vi "Remove Filename Invalid Char.vi"(2 "Input string":string, 6 "Replace Using ...":enum16{"Underscore", "Space"}(ring)) -> (16 "Output String":string)   [LabVIEW 2022 SP3, in "Generic Utilities.lvclass"]
uses:
  Generic Utilities.lvclass
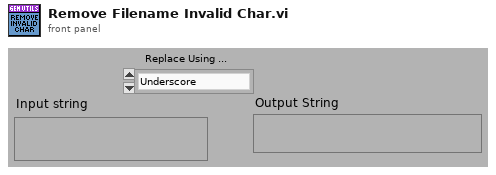
[diagram p1: front panel]
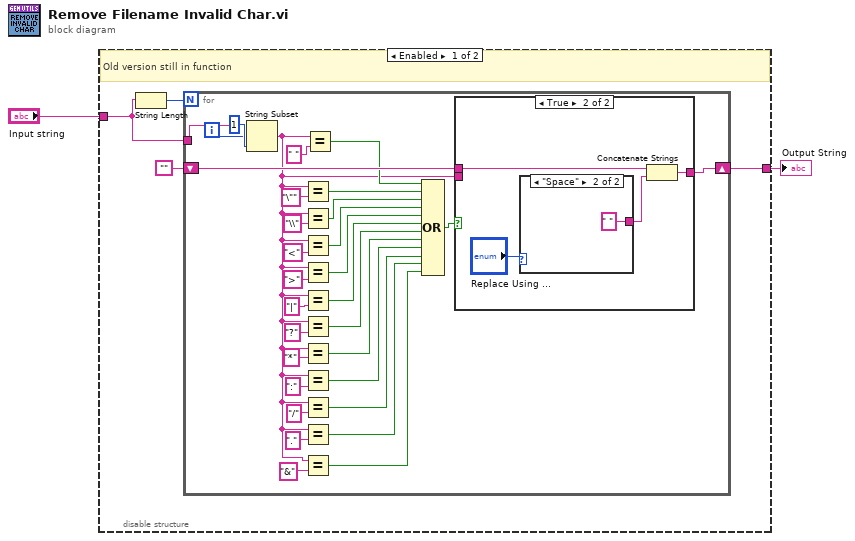
[diagram p0: block diagram]
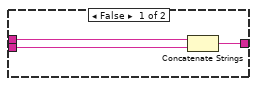
[diagram p2: hidden frame]
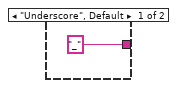
[diagram p3: hidden frame]
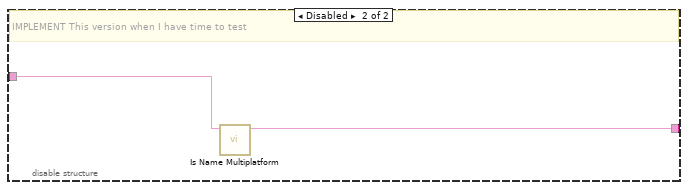
[diagram p4: hidden frame]
diagram:
  n1 = disable-structure shown="Enabled" {
    disable-tunnel: "Input string" -> [w5 w48]
    disable-tunnel: [w3 w47] -> w1
    frame Enabled {
      # "Old version still in function"
      n2 = String Length(string=w5) -> (length=w4:i32)
      n3 = for {
        N: w4 -> [_]
        shift-right: [w33] -> w3
        shift-left: "" -> [w32]
        tunnel: w5 -> [w35]
        i -> [w36]
        n4 = String Subset(string=w35, offset (0)=w36, length (rest)=1) -> (substring=w8:string)
        n5 = Equal?(x=w8, y="\"") -> (x = y?=w21:bool)
        n6 = Equal?(x=w8, y="\\") -> (x = y?=w20:bool)
        n7 = Equal?(x=w8, y="<") -> (x = y?=w19:bool)
        n8 = Equal?(x=w8, y=">") -> (x = y?=w18:bool)
        n9 = Equal?(x=w8, y="|") -> (x = y?=w17:bool)
        n10 = Equal?(x=w8, y="?") -> (x = y?=w16:bool)
        n11 = Equal?(x=w8, y="*") -> (x = y?=w15:bool)
        n12 = Equal?(x=w8, y=":") -> (x = y?=w14:bool)
        n13 = Equal?(x=w8, y="/") -> (x = y?=w13:bool)
        n14 = Equal?(x=w8, y=".") -> (x = y?=w9:bool)
        n15 = Equal?(x=w8, y="&") -> (x = y?=w7:bool)
        n16 = Equal?(x=w8, y=" ") -> (x = y?=w22:bool)
        n17 = Compound Arithmetic op=OR(w22, w21, w20, w19, w18, w17, w16, w15, w14, w13, w9, w7) -> (w12:bool)
        n18 = case shown="True" w12 {
          tunnel: w32 -> [w40 w44]
          tunnel: [w38 w42] -> w33
          tunnel: w8 -> [w39 _]
          frame False {
            n19 = Concatenate Strings(w40, w39) -> (w38:string)
          }
          frame True {
            n20 = case shown="\"Space\"" "Replace Using ..." {
              tunnel: ["_" " "] -> w43
              frame "Underscore", Default {
              }
              frame "Space" {
              }
            }
            n21 = Concatenate Strings(w44, w43) -> (w42:string)
          }
        }
      }
    }
    frame Disabled {
      # "IMPLEMENT This version when I have time to test"
      n22 = call <vilib>:"Is Name Multiplatform.vi"("filename"=w48) -> ("suggested filename"=w47:string)  [unwired: 6 in, 4 out]
    }
  }
  "Output String" <- w1
